vi "GetCollisionParams.vi"(8 "error in (no error)":errorcluster, 11 "GPong in":refnum<class "GPong.lvclass">) -> (0 "error out":errorcluster, 1 "UpDownLeftRightCollide":bool[](array[boolean]), 2 "UpDownLeftRightBounce":dbl[](array[numeric]), 3 "GPong out":refnum<class "GPong.lvclass">)   [LabVIEW 2019, in "RT_Game.lvlib" / "GPong.lvclass"]
uses:
  GPong.lvclass
  Pong/Pong.lvclass
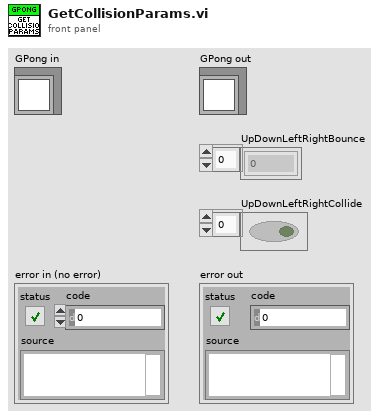
[diagram p1: front panel]
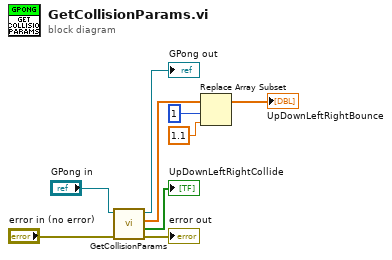
[diagram p0: block diagram]
diagram:
  n1 = call-parent "GetCollisionParams.vi"("error in (no error)"="error in (no error)", "Pong in"="GPong in") -> ("error out"=→"error out":errorcluster, "UpDownLeftRightCollide"=→"UpDownLeftRightCollide":bool[], "UpDownLeftRightBounce"=w7:dbl[], "Pong out"=→"GPong out":refnum<class "GPong.lvclass">)  [unwired: 6 in]
  n2 = Replace Array Subset(array=w7, new element=1.1 ("new element/subarray"), index=1) -> (→"UpDownLeftRightBounce":dbl[])
